vi "SetTarget.vi"(8 "error in (no error)":errorcluster, 9 "Target Rate Limit (T/min)":dbl, 10 "Target Field (T)":dbl[](array[numeric]), 11 "Instrument.VRM in":refnum<class "Instrument.OxfordVRM.lvclass">) -> (0 "error out":errorcluster, 3 "Instrument.VRM out":refnum<class "Instrument.OxfordVRM.lvclass">)   [LabVIEW 2019, in "Instrument.OxfordVRM.lvclass"]
uses:
  Instrument.OxfordVRM.lvclass
  Typedefs/Instrument.VRM.protectedCommands-enum.ctl
  Typedefs/Instrument.VRM.SetTarget--cluster.ctl
  Typedefs/VRM Magnet Axis--Enum.ctl
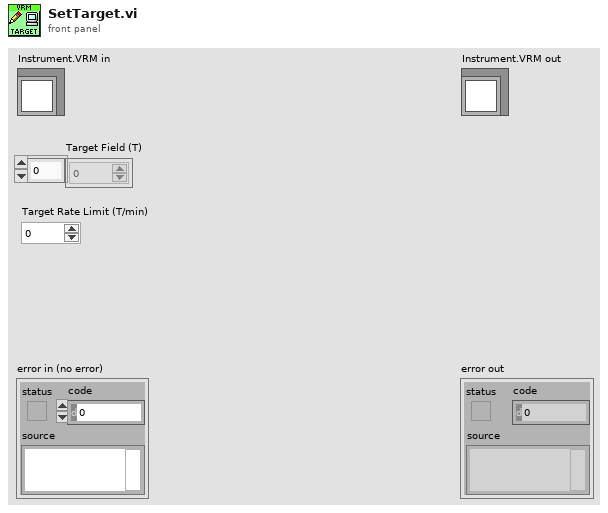
[diagram p1: front panel]
types:
  T1 = typedef "Instrument.OxfordVRM.lvclass/Instrument.VRM.SetTarget--cluster.ctl" = cluster{"field":dbl[], "rate":dbl, "axis":T2}
  T2 = typedef "Instrument.OxfordVRM.lvclass/VRM Magnet Axis--Enum.ctl" = enum16{"X", "Y", "Z", "ALL"}
  T3 = typedef "Instrument.OxfordVRM.lvclass/Instrument.VRM.protectedCommands-enum.ctl" = enum16{"Hold", "RampToSet", "RampToZero", "Clamp", "SetTarget", "GetStatus", "GetTarget", "GetField"}
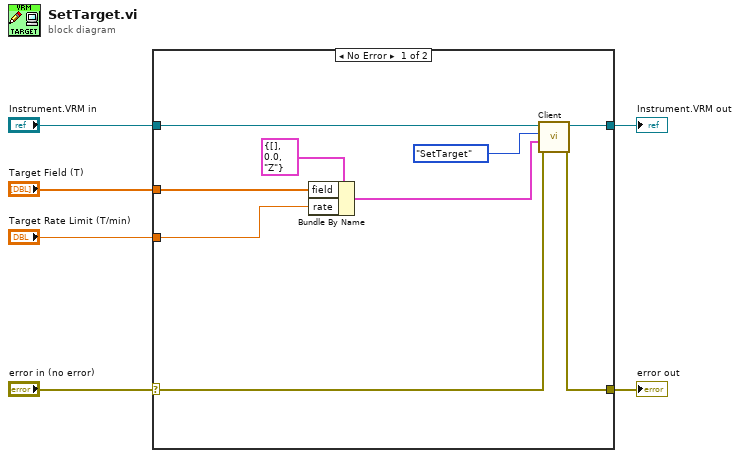
[diagram p0: block diagram]
diagram:
  n1 = case shown="No Error" "error in (no error)" {
    selector: "error in (no error)" -> [w7 w17]
    tunnel: "Target Rate Limit (T/min)" -> [w12 _]
    tunnel: [w8 w17] -> w5
    tunnel: "Target Field (T)" -> [w13 _]
    tunnel: "Instrument.VRM in" -> [w15 w16]
    tunnel: [w14 w16] -> w1
    frame No Error {
      n2 = Bundle By Name(cluster=T1 {"field"=[], "rate"=0.0, "axis"=enum."Z"} ("setTarget"), "field"=w13, "rate"=w12) -> (w11:T1)
      n3 = call-dynamic "Client.vi"("error in (no error)"=w7, "Data in"=w11, "Command in"=Instrument.VRM.protectedCommands-enum."SetTarget" ("protectedCommands"), "Instrument in"=w15) -> ("error out"=w8:errorcluster, "Instrument out"=w14:refnum<class "Instrument.OxfordVRM.lvclass">)  [unwired: 4 in, 2 out]
    }
    frame Error {
    }
  }
  "Instrument.VRM out" <- w1
  "error out" <- w5
